vi "RMS Measurement (Amplitude Reg) Test.vi"() -> ()   [LabVIEW 2014]
uses:
  <vilib>/Platform/TimedLoop/XDataNode/timing_clust.ctl
  <vilib>/Platform/TimedLoop/XDataNode/nitl_modes.ctl
  <vilib>/Platform/TimedLoop/XDataNode/wakeup.ctl
  <vilib>/rvi/FXPMathLib/basic elements/FxpIntAccumulator/subVIs/nifxpmath_IntAccumulator_SimConfig.ctl
  <vilib>/rvi/FXPMathLib/FxpSqrt/subVIs/nifxpmath_Sqrt_SimConfig.ctl
  <vilib>/fxp/LVFixedPointOverflowPolicyTypeDef.ctl
  <vilib>/rvi/Emulation/niFpgaSctlEmulationGetInTimedLoop.vi
  <vilib>/rvi/Emulation/niFpgaEmulationReportErrorSimple.vi
  <vilib>/rvi/Emulation/niFpgaGetClockAttributes.vi
  <vilib>/rvi/Emulation/niFpgaCriticalErrorInLSC.vi
  <vilib>/rvi/Memory/Memory_Emulation/nirvimemoryFastEmulation.vi
  <vilib>/rvi/Memory/Memory_Emulation/nirvimemoryEmulation.vi
  <vilib>/rvi/Emulation/niFpgaEmulationIsFPGAContextNoSignature.vi
  <vilib>/rvi/DataTransferAndStorage/Container/Common/niFpgaContainerGetUniqueNameForEmu.vi
  <vilib>/rvi/Emulation/niFpgaProcessEmulError.vi
  <vilib>/rvi/errors/nirviReportUnexpectedCaseInternalError (U32).vi
  <vilib>/rvi/errors/niFpgaSetErrorForExecOnDevCompSimple.vi
  <vilib>/rvi/eio/common/nirviEmuReportErrorAndStop.vi
  <vilib>/rvi/FIFO/Fifo_Resource/nirvififoEmulationSetSize.vi
  <vilib>/rvi/FIFO/Fifo_Resource/nirviFifoEmulationQueueMgr.vi
  <instcachedir>/0/nirviFifoEmulationQueueMgr_E5CAEC123FF24DC58D834DCA3CDAA9B5.lvgen/nirviFifoEmulationQueueMgr_E5CAEC123FF24DC58D834DCA3CDAA9B5_010.vi
  <vilib>/rvi/FIFO/Fifo_Resource/nirvififoEmulationDetermineInputValidOut.vi
  <vilib>/rvi/FIFO/Fifo_Resource/nirvififoEmulationCreateLock.vi
  <vilib>/rvi/FIFO/Fifo_Resource/nirvififoEmulationObtainLock.vi
  <vilib>/rvi/FIFO/Fifo_Resource/nirvififoEmulationReleaseLock.vi
  <vilib>/rvi/occurrence/nirviWaitOnOccurrenceBase.vi
  <vilib>/rvi/errors/nirviReportUnexpectedCaseInternalError.vi
  <vilib>/rvi/interface/RandomDataEmulation/niFpgaRandomDataHandleErrors.vi
  <vilib>/rvi/Analysis/common/codeGenErrors/XNode/niFpgaXNodeCodeGenErrorHandle.vi
  <vilib>/rvi/FXPMathLib/basic elements/FxpIntAccumulator/simVIs/DllFxpIntAccumulator_sub.vi
  <vilib>/rvi/FXPMathLib/FxpSqrt/simVIs/DllSqrtTemp_sub.vi
  <vilib>/rvi/eio/common/nirviEmuTemplateMethod_errors.vi
  <vilib>/Platform/TimedLoop/XDataNode/XDataNode.xnode
  <vilib>/rvi/DataTransferAndStorage/Container/XNode/niFpgaContainer.xnode
  <vilib>/rvi/FIFO/Fifo_Resource/nirvififoEmulationWrite.vi
  <vilib>/rvi/FIFO/Fifo_Resource/nirvififoEmulationRead.vi
  <vilib>/rvi/interface/RandomDataEmulation/nirviRandomDataFpgaReadWriteTemplate.vi
  <vilib>/rvi/Analysis/measure/dc-rms/XNode/niFpgaDC-RMS.xnode
  <vilib>/rvi/FXPMathLib/FxpMul/XNode/nifxpmath_Multiplier.xnode
  <vilib>/rvi/FXPMathLib/basic elements/FxpIntAccumulator/XNode/nifxpmath_IntAccumulator.xnode
  <vilib>/rvi/FXPMathLib/FxpSqrt/XNode/nifxpmath_Sqrt.xnode
  <vilib>/eio/EIOMethodNode/EIOMethodNode.xnode
  <vilib>/Platform/TimedLoop/XDataNode/XDNodeRunTimeDep.lvlib
  <vilib>/rvi/FXPMathLib/sim/FxpSim.dll
panel:
  in  "Amplitude (0:1)":fxp<+,4,1>=1.0
  out "DC (Mean)":fxp<+/-,12,12>
  out "RMS":fxp<+,12,12>
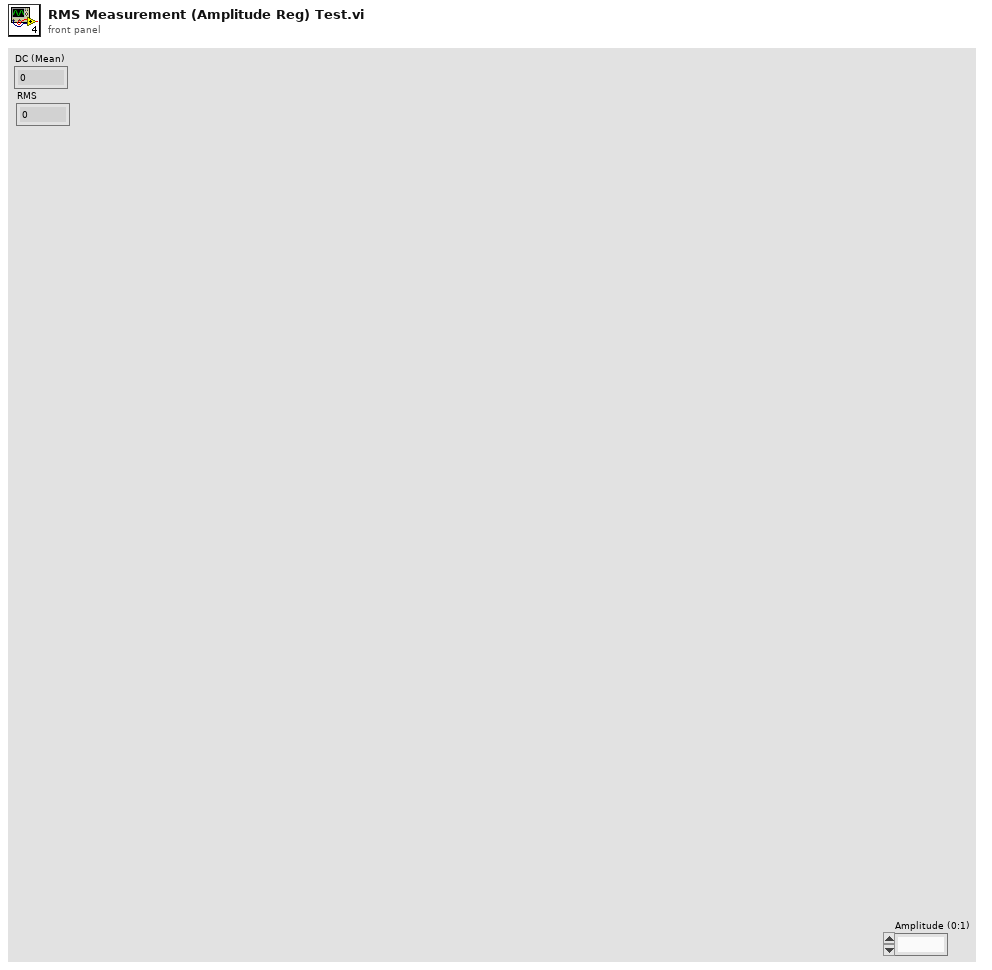
[diagram p1: front panel]
types:
  T1 = typedef "XDNodeRunTimeDep.lvlib/timing_clust.ctl" = cluster{"Expected End [f-1]":u64, "Actual End [f-1]":u64, "Finished Late? [f-1]":bool, "Expected End [i-1]":u64, "Actual End [i-1]":u64, "Finished Late? [i-1]":bool, "Expected Start [i]":u64, "Actual Start [i]":u64, "Expected Start [f]":u64, "Actual Start [f]":u64, "Source Name":string, "Structure Name":string, "Period":i64, "Deadline":i64, "Offset":i64, "Start":i64, "Priority":i32, "Timeout":i32, "Mode":T2, "Wakeup Reason":T3, "Error":errorcluster, "Source Type":string, "Secondary Source Type":string, "Global End Time":u64, "Global Start Time":u64, "Frame Duration":u64, "Iteration Duration":u64, "Assigned CPU":i32, "I/O Scan Engine Mode":u32}
  T2 = typedef "XDNodeRunTimeDep.lvlib/nitl_modes.ctl" = enum32{"No Change", "Process missed periods, maintain original phase", "Discard missed periods, maintain original phase", "Process missed periods, ignore original phase", "Discard missed periods, ignore original phase"}
  T3 = typedef "XDNodeRunTimeDep.lvlib/wakeup.ctl" = enum32{"Normal", "Aborted", "Asynchronous wakeup", "Timing source error", "Timed loop error", "Timeout"}
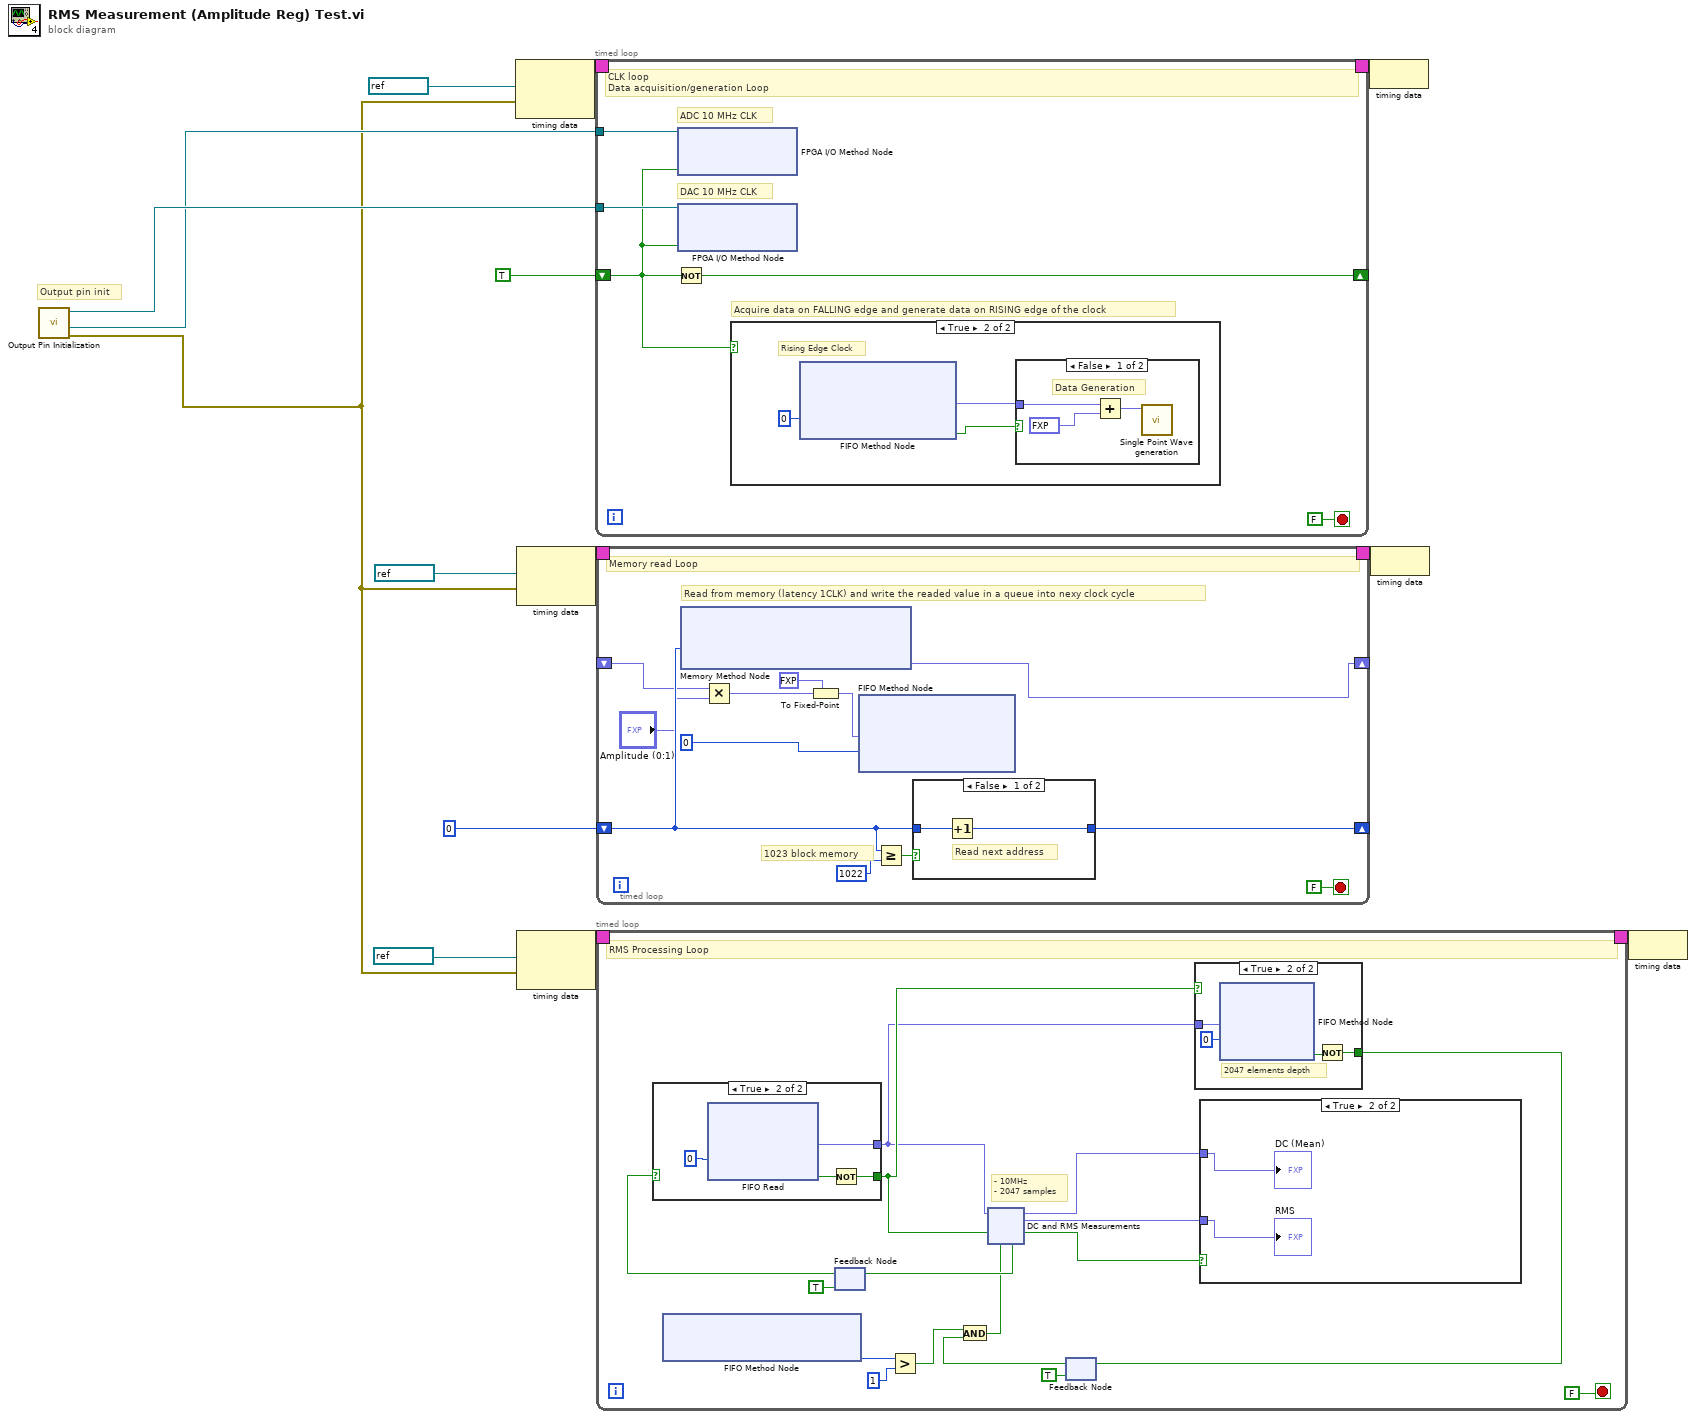
[diagram p0: block diagram]
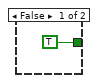
[diagram p2: hidden frame]
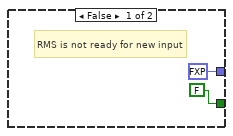
[diagram p4: hidden frame]
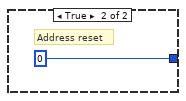
[diagram p5: hidden frame]
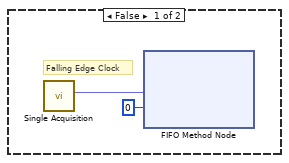
[diagram p6: hidden frame]
diagram:
  # "Output pin init"
  n1 = call "Output Pin Initialization.vi"() -> ("error out"=w1:errorcluster, "I/O Out Clock DAC (pin16)"=w2:refnum<k21>, "I/O Out Clock ADC (pin17)"=w3:refnum<k21>)  [unwired: 8 in]
  n2 = node-c288(refnum<k21> "20MHz" ("Source Name"), w1) -> (w14:T1)
  n3 = node-c288(refnum<k21> "10MHz" ("Source Name"), w1) -> (w12:T1)
  n4 = node-c288(refnum<k21> "10MHz" ("Source Name"), w1) -> (w10:T1)
  n5 = timed-loop {
    timing: w14 -> [_]
    timing-out: [_] -> w13
    shift-right: [w17] -> _
    shift-left: TRUE -> [w15]
    tunnel: w2 -> [w19]
    tunnel: w3 -> [w16]
    stop <- FALSE stop-if-true
    # "DAC 10 MHz CLK"
    # "Acquire data on FALLING edge and generate data on RISING edge of the clock"
    # "ADC 10 MHz CLK"
    # "CLK loop\nData acquisition/generation Loop"
    n6 = Not(x=w15) -> (.not. x?=w17:bool)
    n7 = xnode "FPGA I/O Method Node"("FPGA I/O In"=w19, "Data"=w15) -> ()  [unwired: 1 out]
    n8 = xnode "FPGA I/O Method Node"("FPGA I/O In"=w16, "Data"=w15) -> ()  [unwired: 1 out]
    n9 = case shown="True" w15 {
      frame False {
        # "Falling Edge Clock"
        n10 = call "Single Acquisition.vi"() -> ("Out"=w20:fxp<+/-,12,12>)  [unwired: 10 in, 1 out]
        n11 = xnode ("FIFO Method Node")("Element"=w20, "Timeout"=0) -> ()  [unwired: 1 in, 2 out]
      }
      frame True {
        # "Rising Edge Clock"
        n12 = xnode ("FIFO Method Node")("Timeout"=0) -> ("Element"=w22:fxp<+/-,12,12>, "Timed Out?"=w23:bool)  [unwired: 1 in, 1 out]
        n13 = case shown="False" w23 {
          tunnel: w22 -> [w27 _]
          frame False {
            # "Data Generation"
            n14 = Add(x=w27, y=fxp<+,12,12> 2048.0) -> (x+y=w25:fxp<+/-,14,14>)
            n15 = call "Single Point Wave generation.vi"("Data To Write"=w25) -> ()  [unwired: 10 in, 1 out]
          }
          frame True {
            # "FPGA memory slow"
          }
        }
      }
    }
  }
  n16 = timed-loop {
    timing: w12 -> [_]
    timing-out: [_] -> w11
    shift-right: [w35] -> _
    shift-left: _ -> [w31]
    shift-right: [w39] -> _
    shift-left: u32 0 -> [w36]
    stop <- FALSE stop-if-true
    # "1023 block memory"
    # "Read from memory (latency 1CLK) and write the readed value in a queue into nexy clock cycle"
    # "Memory read Loop"
    n17 = xnode ("Memory Method Node")("Address"=w36) -> ("Data"=w35:fxp<+/-,12,12>)  [unwired: 1 in, 1 out]
    n18 = Multiply(x=w31, y="Amplitude (0:1)") -> (x*y=w32:fxp<+/-,16,13>)
    n19 = To Fixed-Point(fixed-point type=fxp<+/-,12,12> 0.0, number=w32) -> (fixed-point=w30:fxp<+/-,12,12>)
    n20 = xnode ("FIFO Method Node")("Element"=w30, "Timeout"=0) -> ()  [unwired: 1 in, 2 out]
    n21 = Greater Or Equal?(x=w36, y=u32 1022) -> (x >= y?=w40:bool)
    n22 = case shown="False" w40 {
      tunnel: w36 -> [w43 _]
      tunnel: [w42 u32 0] -> w39
      frame False {
        # "Read next address"
        n23 = Increment(x=w43) -> (x+1=w42:u32)
      }
      frame True {
        # "Address reset"
      }
    }
  }
  n24 = timed-loop {
    timing: w10 -> [_]
    timing-out: [_] -> w9
    stop <- FALSE stop-if-true
    # "- 10MHz\n- 2047 samples"
    # "RMS Processing Loop"
    n25 = xnode ("FIFO Method Node")() -> ("Number of Elements to Write"=w53:u32)  [unwired: 1 in, 1 out]
    n26 = feedback #1(TRUE ("ready for input")) -> (w62:bool)
    n27 = case shown="True" w62 {
      tunnel: [FALSE w226] -> w55
      tunnel: [fxp<+/-,12,12> 0.0 ("Element") w223] -> w54
      frame False {
        # "RMS is not ready for new input"
      }
      frame True {
        n28 = xnode ("FIFO Read")("Timeout"=0) -> ("Element"=w223:fxp<+/-,12,12>, "Timed Out?"=w225:bool)  [unwired: 1 in, 1 out]
        n29 = Not(x=w225) -> (.not. x?=w226:bool)
      }
    }
    n30 = Greater?(x=w53, y=u32 1) -> (0:w51:bool)
    n31 = feedback #2(TRUE) -> (w48:bool)
    n32 = And(x=w51, y=w48) -> (x .and. y?=w47:bool)
    n33 = xnode "DC and RMS Measurements"("input data"=w54, "input valid"=w55, "ready for output"=w47) -> ("DC"=w58:fxp<+/-,12,12>, "RMS"=w57:fxp<+,12,12>, "output valid"=w60:bool, "ready for input"=w59:bool)  [unwired: 1 in]
    n34 = feedback-in #1(w59) -> ()
    n35 = case shown="True" w55 {
      tunnel: w54 -> [_ w67]
      tunnel: [TRUE w64] -> w50
      frame False {
      }
      frame True {
        # "2047 elements depth"
        n36 = xnode ("FIFO Method Node")("Element"=w67, "Timeout"=0) -> ("Timed Out?"=w65:bool)  [unwired: 1 in, 1 out]
        n37 = Not(x=w65) -> (.not. x?=w64:bool)
      }
    }
    n38 = feedback-in #2(w50) -> ()
    n39 = case shown="True" w60 {
      tunnel: w58 -> [_ w220]
      tunnel: w57 -> [_ w219]
      frame False {
        # "Output is not valid:\nvalue of DC and RMS\nare not ready"
      }
      frame True {
        "DC (Mean)" <- w220
        "RMS" <- w219
      }
    }
  }
  n40 = node-c288(w13) -> ()
  n41 = node-c288(w11) -> ()
  n42 = node-c288(w9) -> ()
